vi "Read Ball Dumper V.5.0.vi"(11 "Joystick Buttons":bool[](array[boolean])) -> ()   [LabVIEW 2016]
uses:
  Robot Global Data V.5.0.vi
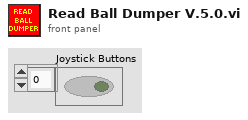
[diagram p1: front panel]
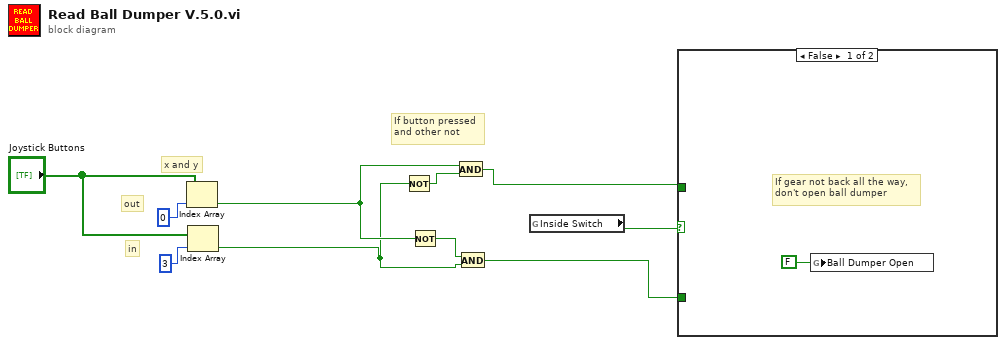
[diagram p0: block diagram]
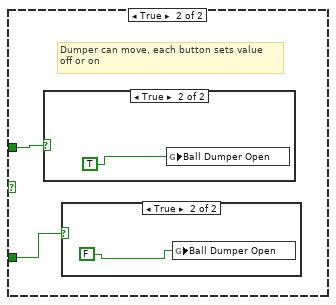
[diagram p2: hidden frame]
diagram:
  # "If button pressed\nand other not"
  # "x and y"
  # "in"
  # "out"
  n1 = Index Array(array="Joystick Buttons", index=0) -> (element=w4:bool)
  n2 = Index Array(array="Joystick Buttons", index=3) -> (element=w3:bool)
  n3 = Not(x=w3) -> (.not. x?=w5:bool)
  n4 = Not(x=w4) -> (.not. x?=w6:bool)
  n5 = And(x=w4, y=w5) -> (x .and. y?=w8:bool)
  n6 = And(x=w6, y=w3) -> (x .and. y?=w7:bool)
  n7 = global read "Robot Global Data V.5.0.vi" "Inside Switch"() -> (w2:bool)
  n8 = case shown="False" w2 {
    tunnel: w8 -> [_ w13]
    tunnel: w7 -> [_ w12]
    frame False {
      # "If gear not back all the way,\ndon't open ball dumper"
      n9 = global write "Robot Global Data V.5.0.vi" "Ball Dumper Open"(FALSE) -> ()
    }
    frame True {
      # "Dumper can move, each button sets value\noff or on"
      n10 = case shown="True" w13 {
        frame False {
        }
        frame True {
          n11 = global write "Robot Global Data V.5.0.vi" "Ball Dumper Open"(TRUE) -> ()
        }
      }
      n12 = case shown="True" w12 {
        frame False {
        }
        frame True {
          n13 = global write "Robot Global Data V.5.0.vi" "Ball Dumper Open"(FALSE) -> ()
        }
      }
    }
  }
